vi "CR-导丝上料一致性检测.vi"(8 "error in (no error)":errorcluster caption="错误输入（无错误）", 11 "名称或相对路径":string="Template Program") -> (0 "error in (no error) 2":errorcluster caption="错误输入（无错误）")   [LabVIEW 2017]
uses:
  Picture/SaveButtom.ctl
  <vilib>/vision/Measure.llb/Straight Edge Options.ctl
  <vilib>/vision/Measure.llb/Straight Edge Process.ctl
  <vilib>/vision/Measure.llb/Edge Options.ctl
  <vilib>/vision/Measure.llb/Edge Polarity.ctl
  Global System.vi
  <vilib>/Utility/xml.llb/Write to XML File(string).vi
panel:
  in  "获取图像":bool
  in  "ROI获取":bool
  in  "创建模板":bool
  in  "保存图像":bool
  out "添加的路径":path
  in  "刷新":bool
  in  "测试按钮":bool
  in  "保存按钮":bool
  in  "Main":enum32{"主参数", "模板匹配参数 ", "位置范围设定", "测试效果"}(tab)
  in  "导丝上料一致性基础参数":T1={"IsNorImage"=TRUE, "Exposure Values"=100289, "ImagePath"=path "C:/Users/hedongpo/Desktop/514-hdp/Alignment Assemble System/Test Picture/B/3.bmp"} caption="参数界面" {"Exposure Values" scale=0.0..200000.0}
  in  "导丝上料一致性参数":T7={"Rectangle"={"Left"=0, "Top"=0, "Right"=0, "Bottom"=0, "Rotation"=0.0}, "Find Straight Edge 1"={"Number of Lines"=1, "Type"=enum."First Edge Rake", "Min. Score"=10.0, "Max. Score"=1000.0, "Orientation"=0.0, "Angle Range"=45.0, "Angle Tolerance"=1.0, "Step Size"=11, "Min. SNR (db)"=0.0, "Min. Points (%)"=25.0, "Hough Iterations"=5}, "Process (Edge Detector 1)"=enum."Get All Edges", "Edge Options (Edge Detector 1)"={"Edge Polarity"=0, "Kernel Size"=9, "Width"=1, "Minimum Edge Strength"=8.0, "Interpolation Type"=enum."Bilinear Fixed", "Data Processing Method"=enum."Average"}, "Options (Find Straight Edge 1)"={"Search Direction"=0, "Edge Options"={"Edge Polarity"=0, "Kernel Size"=3, "Width"=1, "Minimum Edge Strength"=32.0, "Interpolation Type"=enum."Bilinear Fixed", "Data Processing Method"=enum."Average"}, "Show Search Area"=TRUE, "Show Search Lines"=TRUE, "Show Edges Found"=TRUE, "Show Result"=TRUE, "Search Area Color"=65280, "Search Lines Color"=255, "Edge Locations Color"=16776960, "Result Color"=16711680, "Overlay Group Name"=""}, "Parameters (Pattern Matching 1)"={"Number of Matches Requested"=1, "Minimum Match Score"=799.0, "Angle Ranges"=[{"Start Angle"=-180.0, "End Angle"=180.0}, {"Start Angle"=0.0, "End Angle"=360.0}]}, "Template File Path (Pattern Matching 1)"=path "D:/Inspect System/Source Code/Template Program/一致性模板.png"} {"Options (Find Straight Edge 1)"."Search Direction" items=["Left to Right", "Right to Left", "Top to Bottom", "Bottom to Top"]; "Options (Find Straight Edge 1)"."Edge Options"."Edge Polarity" items=["All Edges", "Rising Edges", "Falling Edges"]; "Options (Find Straight Edge 1)"."Edge Options"."Minimum Edge Strength" format="%.2f"; "Options (Find Straight Edge 1)"."Edge Options"."Width" step=2; "Options (Find Straight Edge 1)"."Edge Options"."Kernel Size" step=2; "Edge Options (Edge Detector 1)"."Edge Polarity" items=["All Edges", "Rising Edges", "Falling Edges"]; "Find Straight Edge 1"."Min. Points (%)" min=0.0 max=100.0; "Find Straight Edge 1"."Min. SNR (db)" min=0.0; "Find Straight Edge 1"."Max. Score" min=0.0 max=1024.0; "Find Straight Edge 1"."Min. Score" min=0.0 max=1024.0 step=1.0; "Rectangle"."Rotation" format="%.2f"; "Rectangle"."Left" scale=0.0..1024.0; "Rectangle"."Right" scale=0.0..1024.0}
  in  "位置范围设定":T8={"位置1"={"上限"=726.0, "下限"=686.0}, "位置2"={"上限"=874.0, "下限"=834.0}, "位置3"={"上限"=997.0, "下限"=957.0}, "位置4"={"上限"=1139.0, "下限"=1099.0}, "位置5"={"上限"=1283.0, "下限"=1243.0}, "位置6"={"上限"=1429.0, "下限"=1389.0}, "位置7"={"上限"=1576.0, "下限"=1536.0}, "位置8"={"上限"=1728.0, "下限"=1688.0}, "位置9"={"上限"=1879.0, "下限"=1839.0}, "位置10"={"上限"=2036.0, "下限"=1996.0}}
  out "原始图像":T9(plugin-control)
  out "模板图片":T9(plugin-control)
  out "一致性结果字符串":string
  out "数字":i32
  out "动态范围":sgl[](array[numeric])
  out "路径输出":path
  in  "Vision Paramter Save Buttom":T10
  out "system time":string
  in  "取消按钮":bool
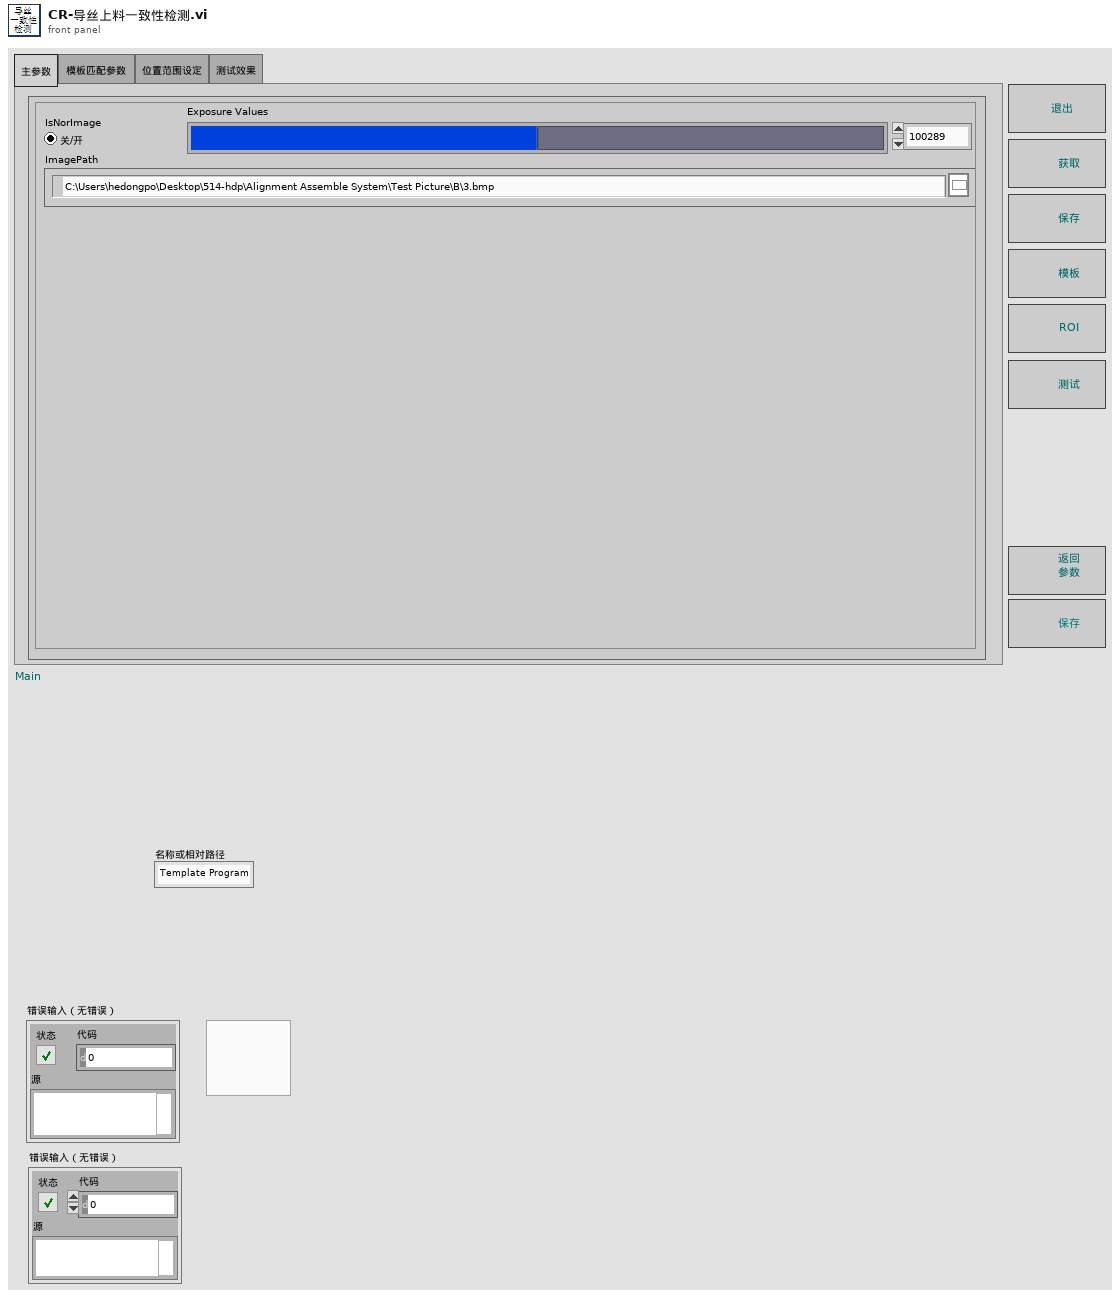
[diagram p1: front panel]
types:
  T1 = cluster{"IsNorImage":bool, "Exposure Values":u32, "ImagePath":path}
  T2 = typedef "IMAQ Rectangle" = cluster{"Left":i32, "Top":i32, "Right":i32, "Bottom":i32, "Rotation":dbl}
  T3 = typedef "Straight Edge Options.ctl" = cluster{"Number of Lines":i32, "Type":T4, "Min. Score":dbl, "Max. Score":dbl, "Orientation":dbl, "Angle Range":dbl, "Angle Tolerance":dbl, "Step Size":u32, "Min. SNR (db)":dbl, "Min. Points (%)":dbl, "Hough Iterations":i32}
  T4 = typedef "Straight Edge Process.ctl" = enum32{"First Edge Rake", "Best Edge Rake", "Hough Edge Rake", "First Edge Projection", "Best Edge Projection"}
  T5 = typedef "Edge Options.ctl" = cluster{"Edge Polarity":T6, "Kernel Size":u32, "Width":u32, "Minimum Edge Strength":sgl, "Interpolation Type":enum32{"Zero Order", "Bilinear", "Quadratic", "Cubic", "Bilinear Fixed"}, "Data Processing Method":enum32{"Average", "Median"}}
  T6 = typedef "Edge Polarity.ctl" = u32
  T7 = cluster{"Rectangle":T2, "Find Straight Edge 1":T3, "Process (Edge Detector 1)":enum16{"Get First Edge", "Get First + Last Edge", "Get All Edges", "Get Best Edge"}, "Edge Options (Edge Detector 1)":cluster{"Edge Polarity":u32, "Kernel Size":u32, "Width":u32, "Minimum Edge Strength":sgl, "Interpolation Type":enum32{"Zero Order", "Bilinear", "Quadratic", "Cubic", "Bilinear Fixed"}, "Data Processing Method":enum32{"Average", "Median"}}, "Options (Find Straight Edge 1)":cluster{"Search Direction":u32, "Edge Options":T5, "Show Search Area":bool, "Show Search Lines":bool, "Show Edges Found":bool, "Show Result":bool, "Search Area Color":u32, "Search Lines Color":u32, "Edge Locations Color":u32, "Result Color":u32, "Overlay Group Name":string}, "Parameters (Pattern Matching 1)":cluster{"Number of Matches Requested":i32, "Minimum Match Score":sgl, "Angle Ranges":cluster{"Start Angle":sgl, "End Angle":sgl}[]}, "Template File Path (Pattern Matching 1)":path}
  T8 = cluster{"位置1":cluster{"上限":dbl, "下限":dbl}, "位置2":cluster{"上限":dbl, "下限":dbl}, "位置3":cluster{"上限":dbl, "下限":dbl}, "位置4":cluster{"上限":dbl, "下限":dbl}, "位置5":cluster{"上限":dbl, "下限":dbl}, "位置6":cluster{"上限":dbl, "下限":dbl}, "位置7":cluster{"上限":dbl, "下限":dbl}, "位置8":cluster{"上限":dbl, "下限":dbl}, "位置9":cluster{"上限":dbl, "下限":dbl}, "位置10":cluster{"上限":dbl, "下限":dbl}}
  T9 = typedef "IMAQ Image.ctl" = refnum<image>
  T10 = typedef "SaveButtom.ctl" = bool
  T11 = cluster{"index":i32, "this vi":refnum<vi>, "error out":errorcluster}
  T12 = cluster{"master data":string, "priority":u16, "secondary data":string[]}
  T13 = cluster{"case name":string[], "queue array":refnum<queue>[]}
  T14 = typedef "Image Type" = u32
  T15 = typedef "IMAQdx.ctl" = refnum<k21>
  T16 = cluster{"Global Rectangle":i32[], "Contours":cluster{"Contour Type":u32, "ROI Type":u32, "Points":i32[]}[]}
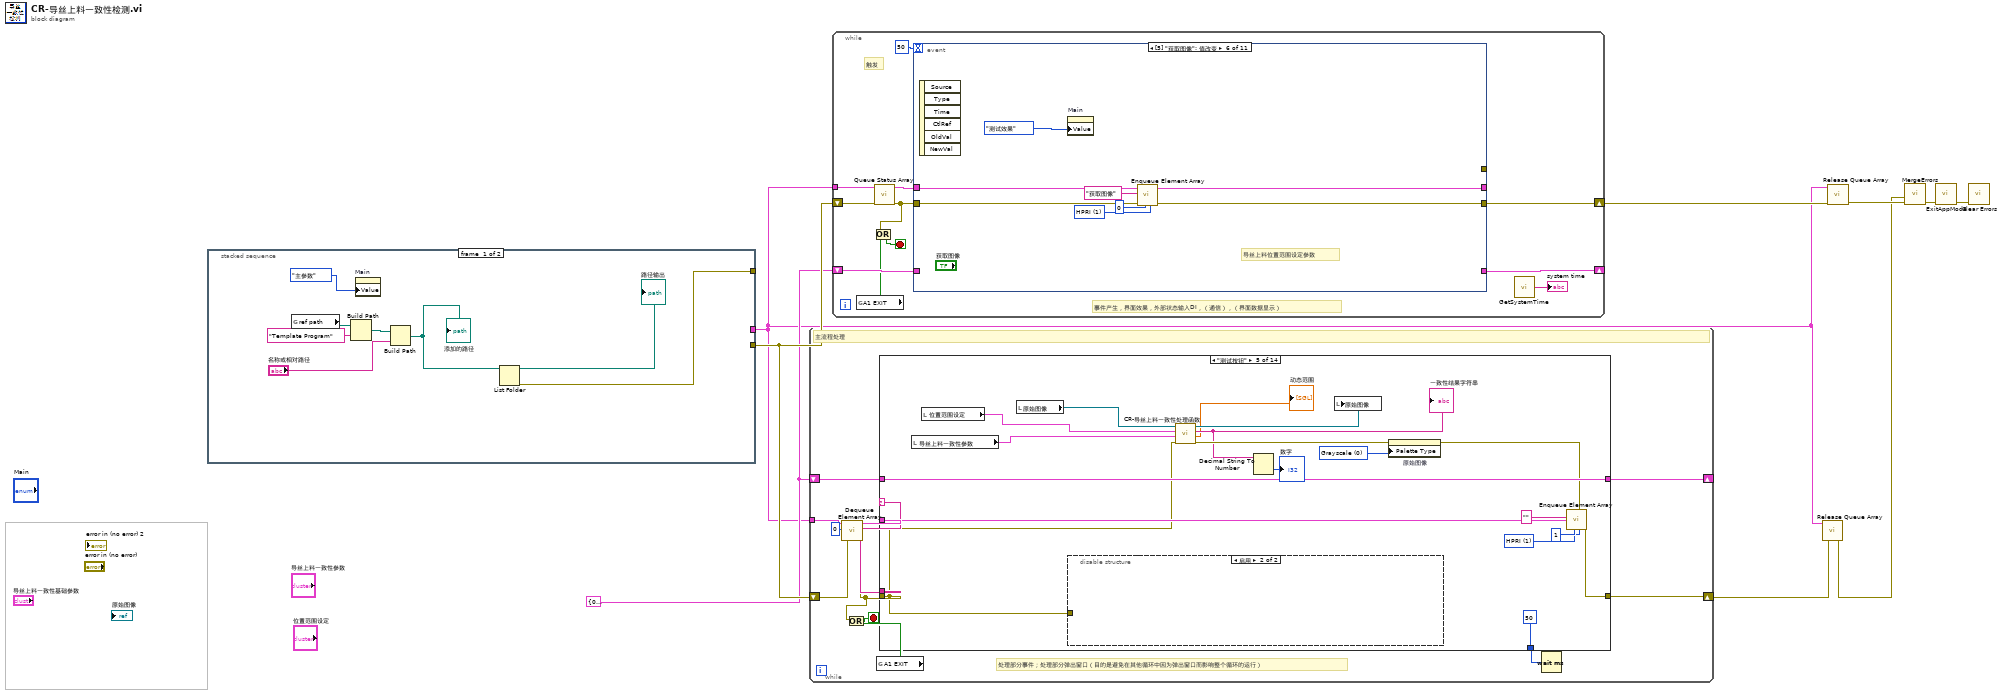
[diagram p0: block diagram]
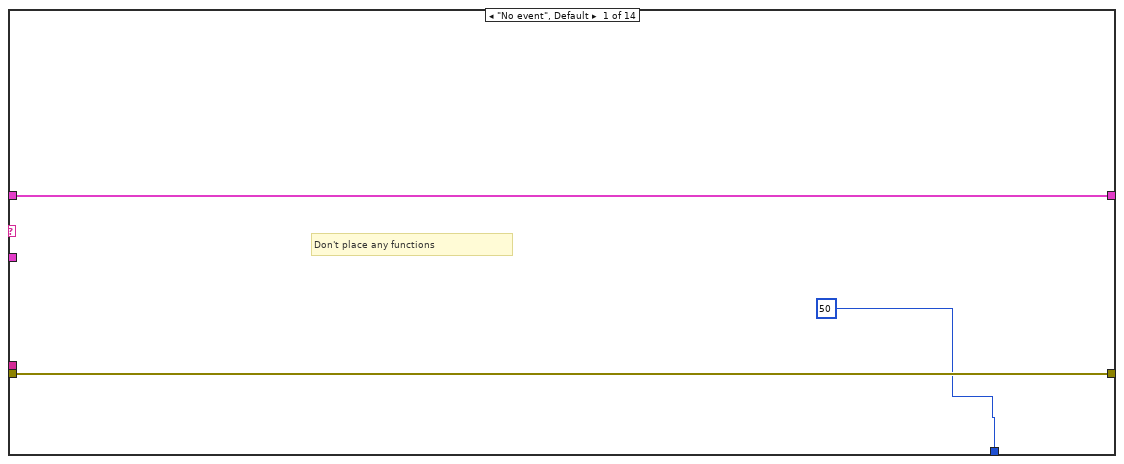
[diagram p2: hidden frame]
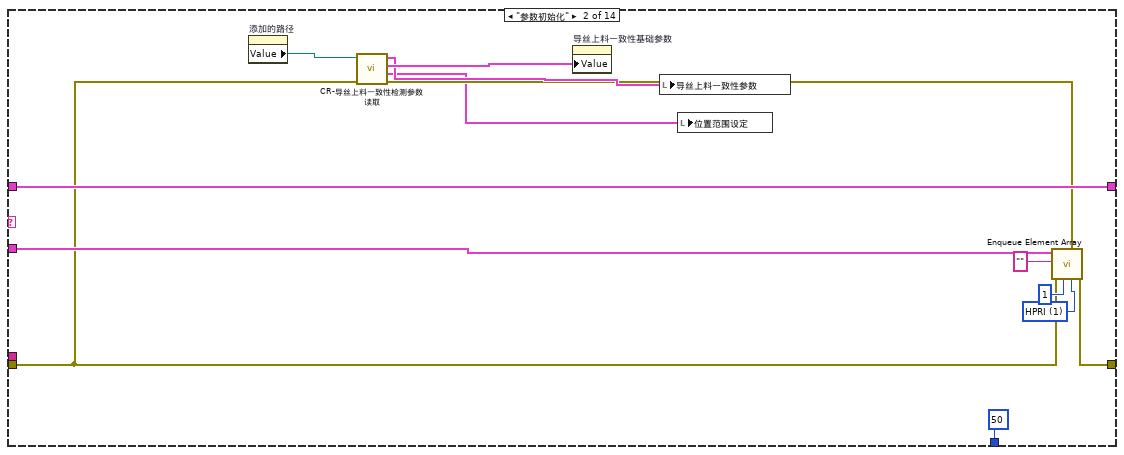
[diagram p3: hidden frame]
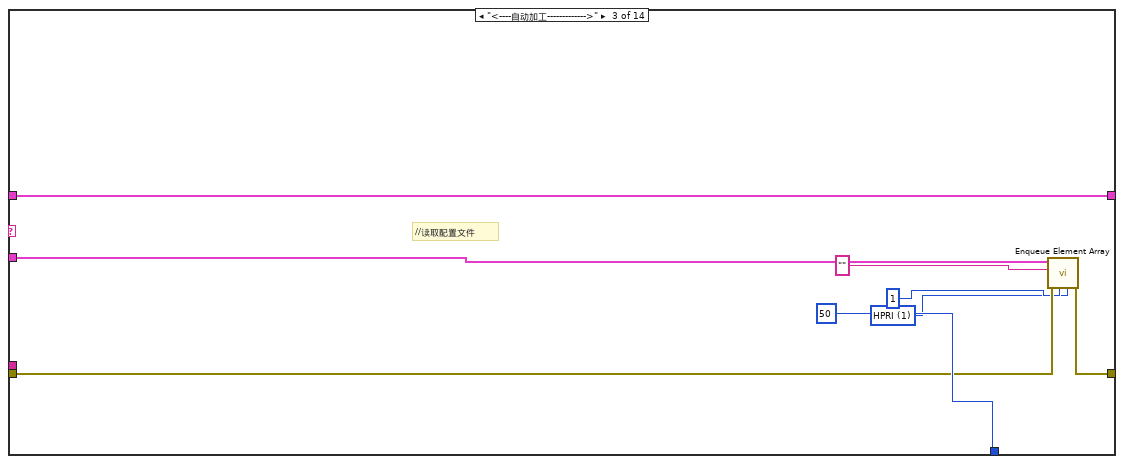
[diagram p4: hidden frame]
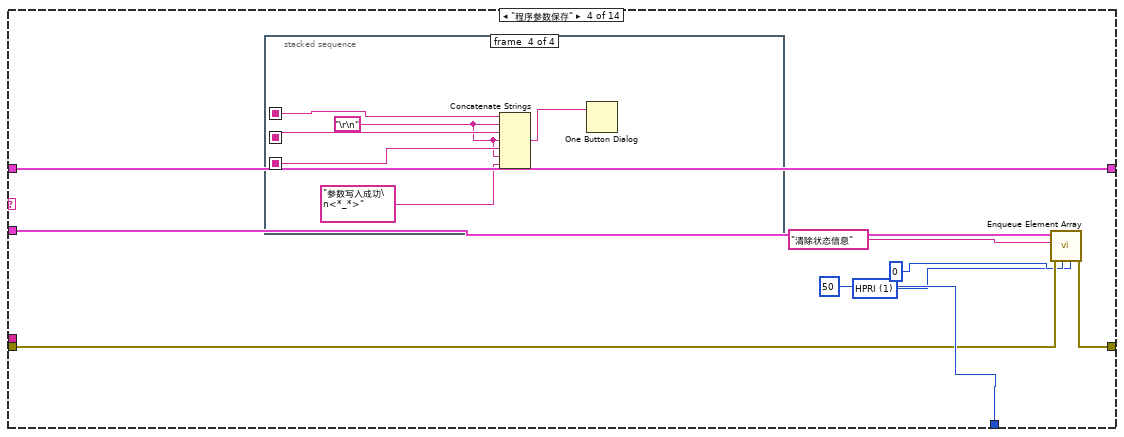
[diagram p5: hidden frame]
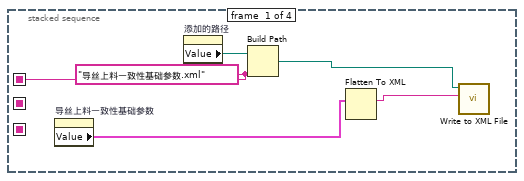
[diagram p6: hidden frame]
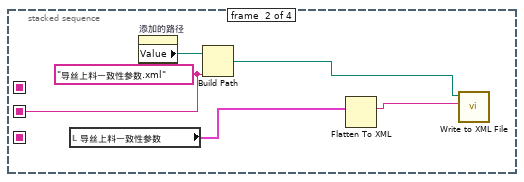
[diagram p7: hidden frame]
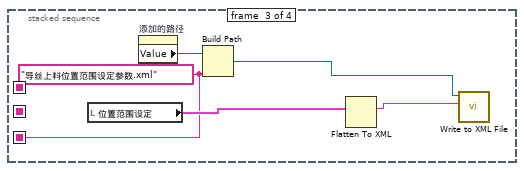
[diagram p8: hidden frame]
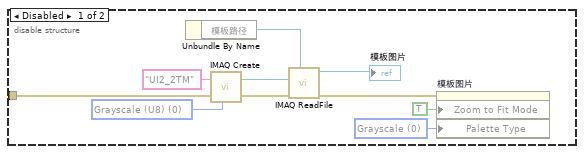
[diagram p9: hidden frame]
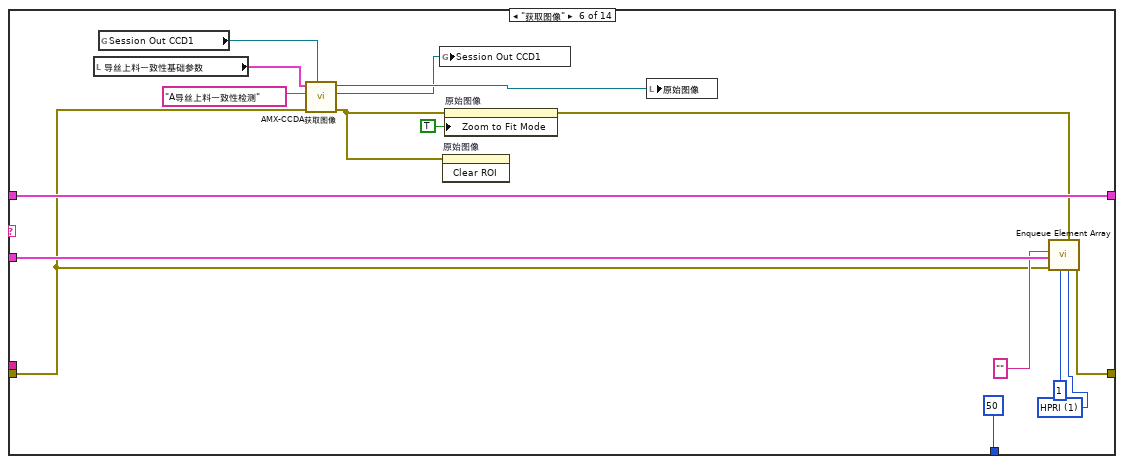
[diagram p10: hidden frame]
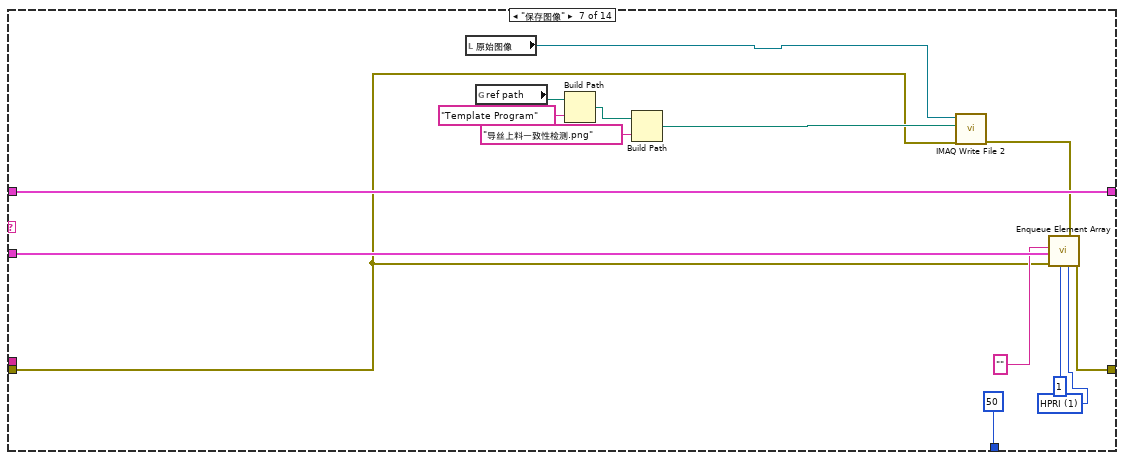
[diagram p11: hidden frame]
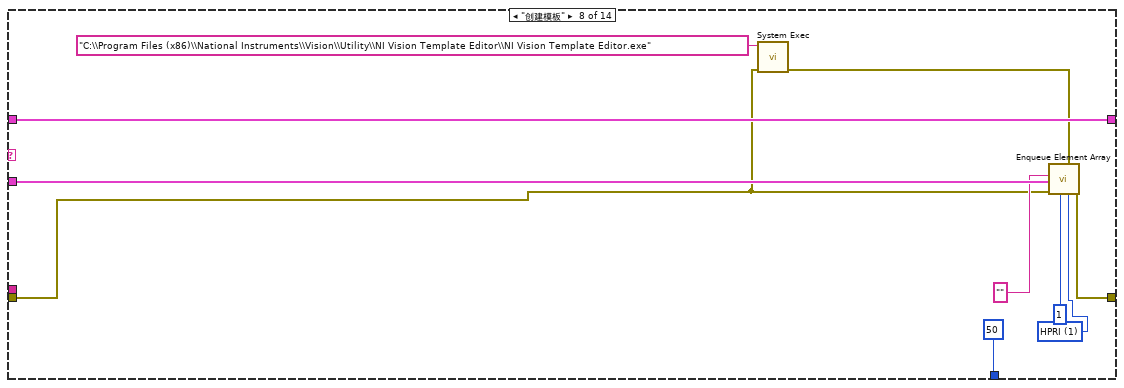
[diagram p12: hidden frame]
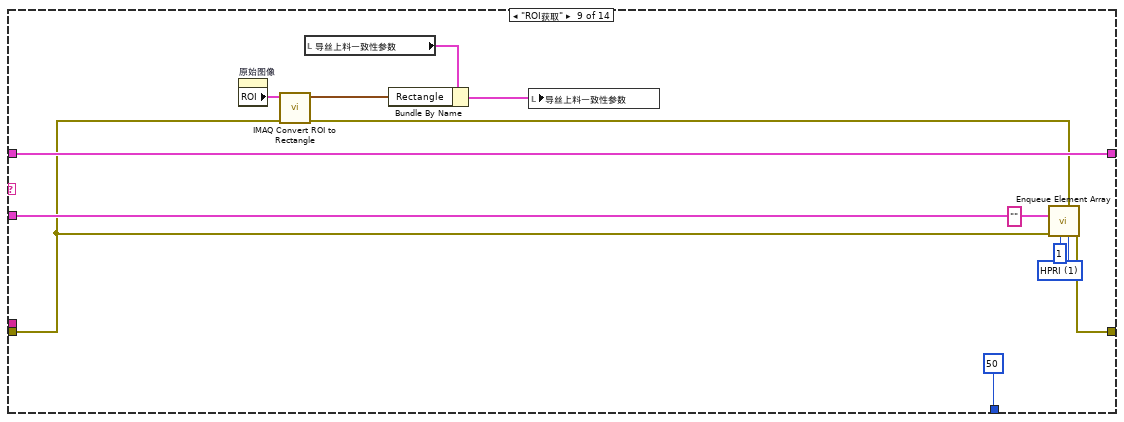
[diagram p13: hidden frame]
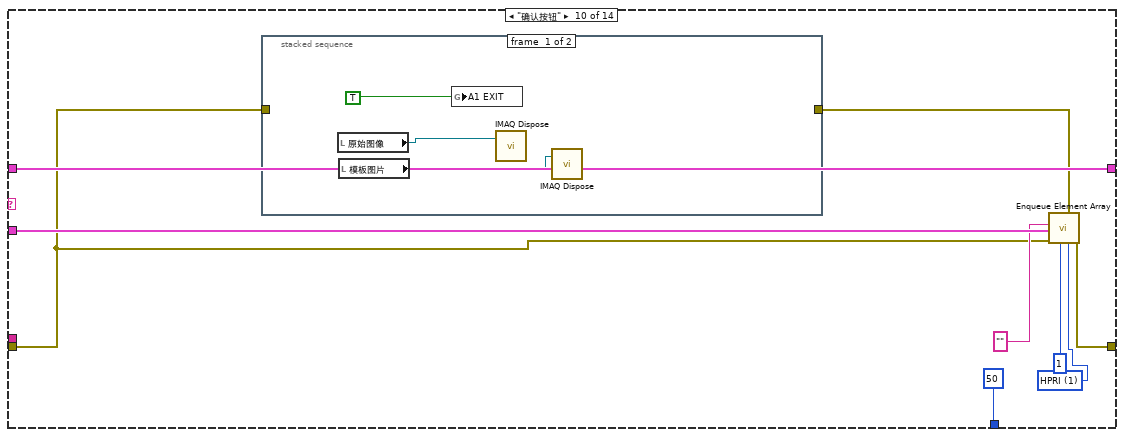
[diagram p14: hidden frame]
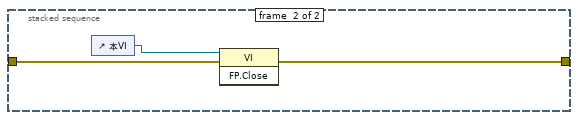
[diagram p15: hidden frame]
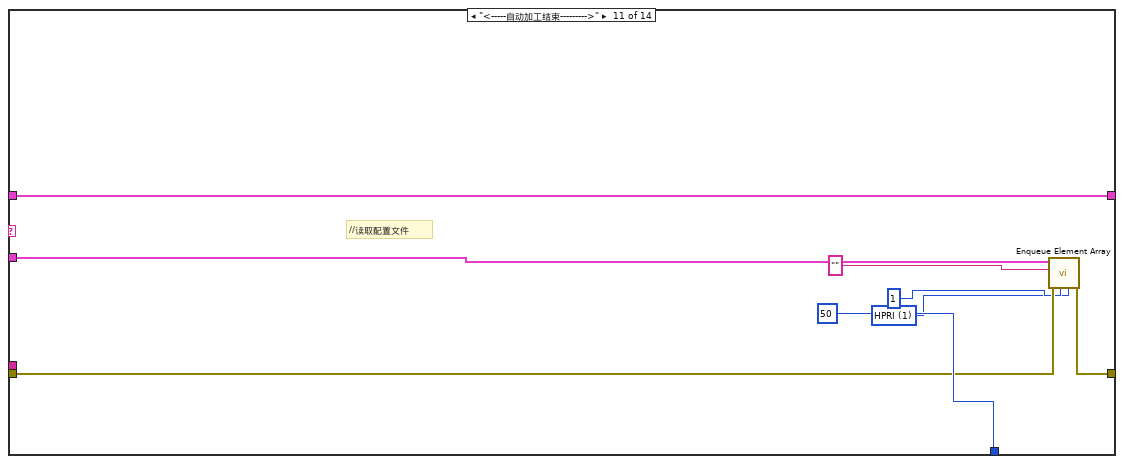
[diagram p16: hidden frame]
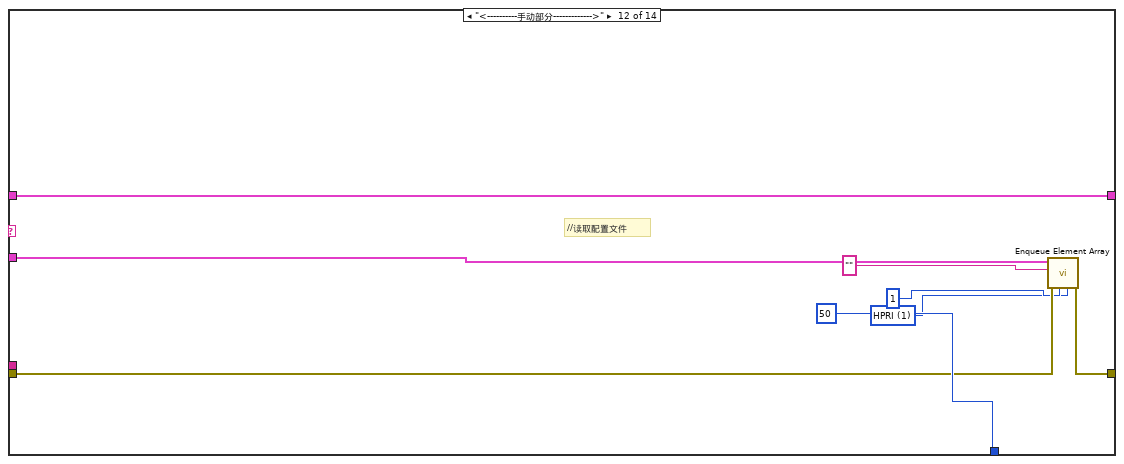
[diagram p17: hidden frame]
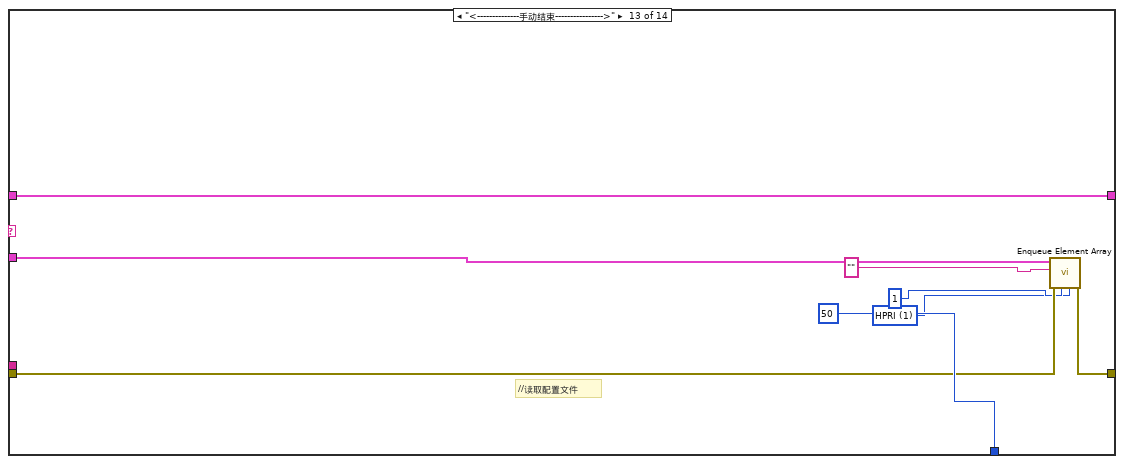
[diagram p18: hidden frame]
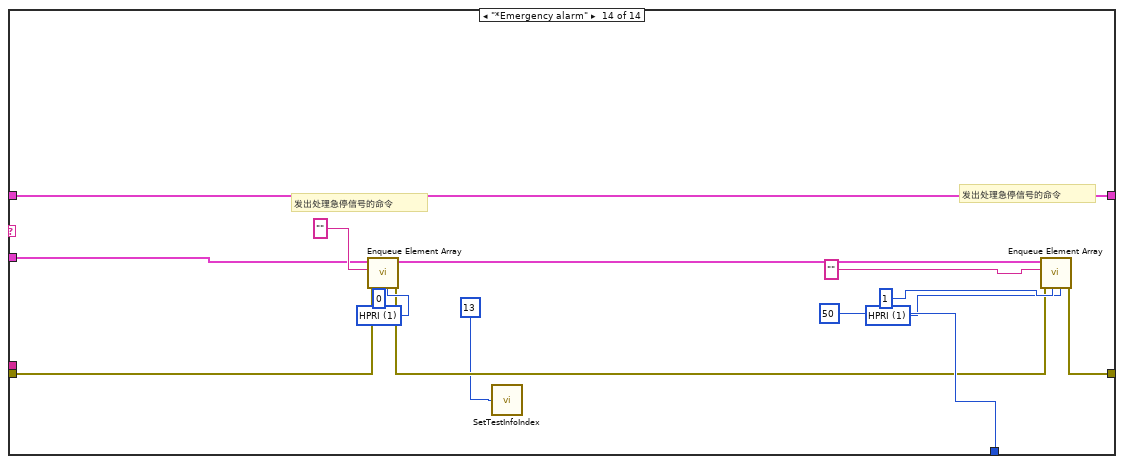
[diagram p19: hidden frame]
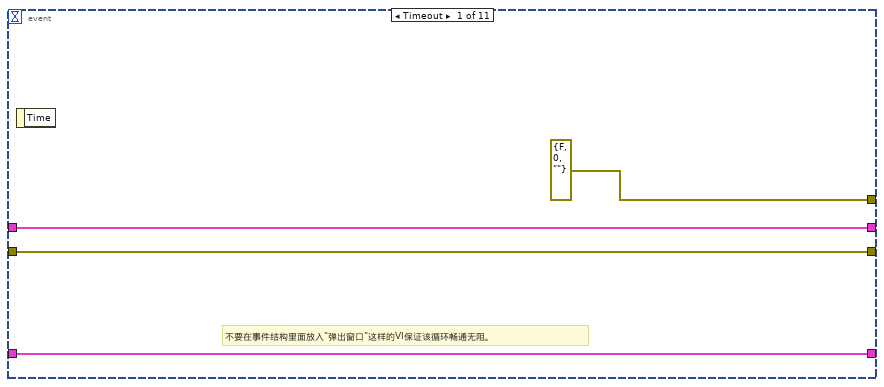
[diagram p20: hidden frame]
diagram:
  w4 = T11 {"index"=0, "this vi"=refnum, "error out"={"status"=FALSE, "code"=0, "source"=""}} ("parameter buffer")
  n1 = stacked-sequence {
    tunnel: [w15 _] -> _
    tunnel: [_ w19] -> w5
    tunnel: [_ w18] -> w1
    frame #0 {
      n2 = global read "Global System.vi" "ref path"() -> (w13:path)
      n3 = Build Path(base path=w13, name or relative path="Template Program" ("名称或相对路径")) -> (appended path=w11:path)
      n4 = property on="Main" class="TabCtl (严格)"("Value"=enum32{"主参数", "模板匹配参数 ", "位置范围设定", "测试效果"}."主参数" ("Main")) -> ()  [unwired: 2 in, 2 out]
      n5 = Build Path(base path=w11, name or relative path="名称或相对路径") -> (appended path=w17:path)
      "添加的路径" <- w17
      n6 = List Folder(path=w17) -> (path out=→"路径输出":path, error out=w15:errorcluster)  [unwired: 3 in, 2 out]
    }
    frame #1 {
      w27 = string[] ["comm queue1", "data queue 11", "data queue 12", "data queue 13", "data queue 14"]  # queue name
      w28 = 4  # queue num
      w29 = T12 {"master data"="", "priority"=0, "secondary data"=[]}  # element data type
      n7 = call "Obtain Queue Array.vi"("queue name"=w27, "element data type"=w29, "queue num"=w28) -> ("error out"=w23:errorcluster, "queue out"=w24:T13)  [unwired: 2 in, 1 out]
      n8 = call "Enqueue Element Array.vi"("queue index"=0, "error in"=w23, "master data"="参数初始化", "queue in"=w24) -> ("error out"=w22:errorcluster, "queue out"=w21:T13)  [unwired: 6 in]
      n9 = disable-structure shown="启用" {
        disable-tunnel: w22 -> [w35 w36]
        disable-tunnel: w21 -> [w34 w37]
        disable-tunnel: "Loading Variable" ("master data") -> [w33 _]
        disable-tunnel: [w31 w36] -> w19
        disable-tunnel: [w30 w37] -> w18
        frame Disabled {
          n10 = call "Enqueue Element Array.vi"("queue index"=12, "error in"=w35, "master data"=w33, "queue in"=w34) -> ("error out"=w31:errorcluster, "queue out"=w30:T13)  [unwired: 6 in]
        }
        frame Enabled {
        }
      }
    }
  }
  n11 = while {
    shift-right: [w50] -> w3
    shift-left: w5 -> [w41]
    shift-right: [w47] -> _
    shift-left: w4 -> [w48]
    tunnel: w1 -> [w43]
    stop <- w38 stop-if-true
    # "处理部分事件；处理部分弹出窗口（目的是避免在其他循环中因为弹出窗口而影响整个循环的运行）"
    # "主流程处理"
    n12 = call "Dequeue Element Array.vi"("queue in"=w43, "queue index"=0, "error in"=w41) -> ("queue out"=w46:T13, "master data"=w45:string, "secondary data"=w44:string[], "error out"=w40:errorcluster)  [unwired: 2 in, 1 out]
    n13 = global read "Global System.vi" "A1 EXIT"() -> (w39:bool)
    n14 = Or(x=w40, y=w39) -> (x .or. y?=w38:bool)
    n15 = case shown="\"测试按钮\"" w45 {
      tunnel: w46 -> [_ w65 w73 w75 w120 w146 w161 w171 w184 w193 w207 w215 w223 w229]
      tunnel: w40 -> [w52 w58 w69 w79 w114 w138 w148 w164 w177 w187 w203 w211 w219 w226]
      tunnel: [w52 w64 w72 w81 w119 w145 w160 w170 w183 w192 w206 w214 w222 w237] -> w50
      tunnel: [50 50 50 50 50 50 50 50 50 50 50 50 50 50] -> w49
      tunnel: w48 -> [w53 w60 w70 w76 w115 w141 w156 w166 w179 w188 w204 w212 w220 w235]
      tunnel: [w53 w60 w70 w76 w115 w141 w156 w166 w179 w188 w204 w212 w220 w235] -> w47
      tunnel: w44 -> [_ _ _ _ _ _ _ _ _ _ _ _ _ _]
      frame "No event", Default {
        # "Don't place any functions"
      }
      frame "参数初始化" {
        w61 = u16 1 items=["HPRI"=1, "LPRI"=0] ("priority")
        n16 = property on="添加的路径" class="Path"() -> ("Value"=w59:path)  [unwired: 2 in, 2 out]
        n17 = call "CR-导丝上料一致性检测参数读取.vi"("error in (no error)"=w58, "基路径"=w59) -> ("error out"=w55:errorcluster, "CR位置范围设定"=w54:T8, "导丝上料一致性基础参数"=w57:T1, "CR导丝上料一致性参数"=w56:T7)  [unwired: 5 in]
        n18 = property on="导丝上料一致性基础参数" class="Clust (严格)"("Value"=w57) -> ()  [unwired: 2 in, 2 out]
        n19 = local write "导丝上料一致性参数"(w56) -> ()
        n20 = local write "位置范围设定"(w54) -> ()
        n21 = call "Enqueue Element Array.vi"("priority"=w61, "device error in"=w55, "queue index"=1, "error in"=w58, "master data"="" ("Element 1"), "queue in"=w65) -> ("error out"=w64:errorcluster)  [unwired: 4 in, 1 out]
      }
      frame "<----自动加工------------->" {
        w67 = u16 1 items=["HPRI"=1, "LPRI"=0] ("priority")
        # "//读取配置文件"
        n22 = call "Enqueue Element Array.vi"("priority"=w67, "queue index"=1, "error in"=w69, "master data"="" ("Element 1"), "queue in"=w73) -> ("error out"=w72:errorcluster)  [unwired: 5 in, 1 out]
      }
      frame "程序参数保存" {
        w77 = u16 1 items=["HPRI"=1, "LPRI"=0] ("priority")
        n23 = stacked-sequence {
          seq-local: [w83 _ _ _] -> [_ _ _ w102]
          seq-local: [_ w89 _ _] -> [_ _ _ w100]
          seq-local: [_ _ w93 _] -> [_ _ _ w99]
          frame #0 {
            w83 = "导丝上料一致性基础参数.xml" ("名称或相对路径")
            n24 = property on="导丝上料一致性基础参数" class="Clust (严格)"() -> ("Value"=w86:T1)  [unwired: 2 in, 2 out]
            n25 = property on="添加的路径" class="Path"() -> ("Value"=w87:path)  [unwired: 2 in, 2 out]
            n26 = Build Path(base path=w87, name or relative path=w83) -> (appended path=w84:path)
            n27 = Flatten To XML(anything=w86) -> (xml string=w85:string)
            n28 = call-poly <vilib>:"Write to XML File.vi"("XML Input"=w85, "XML File Path"=w84) -> ()  [unwired: 7 in, 3 out]
          }
          frame #1 {
            w89 = "导丝上料一致性参数.xml" ("名称或相对路径")
            n29 = local read "导丝上料一致性参数"() -> (w88:T7)
            n30 = property on="添加的路径" class="Path"() -> ("Value"=w92:path)  [unwired: 2 in, 2 out]
            n31 = Build Path(base path=w92, name or relative path=w89) -> (appended path=w90:path)
            n32 = Flatten To XML(anything=w88) -> (xml string=w91:string)
            n33 = call-poly <vilib>:"Write to XML File.vi"("XML Input"=w91, "XML File Path"=w90) -> ()  [unwired: 7 in, 3 out]
          }
          frame #2 {
            w93 = "导丝上料位置范围设定参数.xml" ("名称或相对路径")
            n34 = local read "位置范围设定"() -> (w94:T8)
            n35 = property on="添加的路径" class="Path"() -> ("Value"=w97:path)  [unwired: 2 in, 2 out]
            n36 = Build Path(base path=w97, name or relative path=w93) -> (appended path=w95:path)
            n37 = Flatten To XML(anything=w94) -> (xml string=w96:string)
            n38 = call-poly <vilib>:"Write to XML File.vi"("XML Input"=w96, "XML File Path"=w95) -> ()  [unwired: 7 in, 3 out]
          }
          frame #3 {
            w98 = "\r\n"
            n39 = Concatenate Strings(w102, w98, w100, w98, w99, w98, "参数写入成功\n<*_*>" ("消息")) -> (w101:string)
            n40 = One Button Dialog(message=w101) -> ()  [unwired: 1 in, 1 out]
          }
        }
        n41 = call "Enqueue Element Array.vi"("priority"=w77, "queue index"=0, "error in"=w79, "master data"="清除状态信息" ("Element 1"), "queue in"=w75) -> ("error out"=w81:errorcluster)  [unwired: 5 in, 1 out]
      }
      frame "测试按钮" {
        w110 = u32 0 items=["Grayscale", "Binary", "Gradient", "Rainbow", "Temperature", "User Defined", "Binary 16 Bit", "Gradient 16 Bit", "Rainbow 16 Bit", "Temperature 16 Bit", "User Defined 16 Bit"] ("Palette:Palette Type")
        w116 = u16 1 items=["HPRI"=1, "LPRI"=0] ("priority")
        n42 = local read "导丝上料一致性参数"() -> (w107:T7)
        n43 = local read "位置范围设定"() -> (w108:T8)
        n44 = local read "原始图像"() -> (w112:T9)
        n45 = disable-structure shown="启用" {
          disable-tunnel: w114 -> [w131 _]
          frame Disabled {
            w123 = u32 0 items=["Grayscale", "Binary", "Gradient", "Rainbow", "Temperature", "User Defined", "Binary 16 Bit", "Gradient 16 Bit", "Rainbow 16 Bit", "Temperature 16 Bit", "User Defined 16 Bit"] ("Palette:Palette Type")
            w129 = T14 0 items=["Grayscale (U8)", "Grayscale (I16)", "Grayscale (SGL)", "Complex (CSG)", "RGB (U32)", "HSL (U32)", "RGB (U64)", "Grayscale (U16)"] ("Image Type")
            n46 = Unbundle By Name() -> ("模板路径"=w122:path)  [unwired: 1 in]
            n47 = call "IMAQ Create"("Image Name"="UI2_2TM", "Image Type"=w129, "error in (no error)"=w131) -> ("New Image"=w128:T9, "error out"=w127:errorcluster)  [unwired: 2 in]
            n48 = call "IMAQ ReadFile"("File Path"=w122, "error in (no error)"=w127, "Image"=w128) -> ("error out"=w125:errorcluster, "Image Out"=→"模板图片":T9)  [unwired: 4 in, 3 out]
            n49 = property on="模板图片" class="ImageControl"(error in=w125, "Zoom to Fit Mode"=TRUE, "Palette Type"=w123) -> ()  [unwired: 1 in, 2 out]
          }
          frame Enabled {
          }
        }
        n50 = call "CR-导丝上料一致性处理函数.vi"("error in (no error)"=w114, "导丝上料一致性参数"=w107, "位置范围设定"=w108, "Image in"=w112) -> ("error out"=w111:errorcluster, "动态范围"=→"动态范围":sgl[], "一致性结果字符串"=w106:string, "Image out"=w113:T9)  [unwired: 4 in]
        "一致性结果字符串" <- w106
        n51 = Decimal String To Number(string=w106) -> (number=→"数字":i32)  [unwired: 2 in, 1 out]
        n52 = local write "原始图像"(w113) -> ()
        n53 = property on="原始图像" class="ImageControl"(error in=w111, "Palette Type"=w110) -> (error out=w109:errorcluster)  [unwired: 1 in, 1 out]
        n54 = call "Enqueue Element Array.vi"("priority"=w116, "device error in"=w109, "queue index"=1, "master data"="" ("Element 1"), "queue in"=w120) -> ("error out"=w119:errorcluster)  [unwired: 5 in, 1 out]
      }
      frame "获取图像" {
        w142 = u16 1 items=["HPRI"=1, "LPRI"=0] ("priority")
        n55 = local read "导丝上料一致性基础参数"() -> (w132:T1)
        n56 = global read "Global System.vi" "Session Out CCD1"() -> (w134:T15)
        n57 = call "AMX-CCDA获取图像.vi"("Session Out CCD2"=w134, "error in (no error)"=w138, "Image Name"="A导丝上料一致性检测", "ParamsUI"=w132) -> ("error out"=w135:errorcluster, "Session Out"=w133:T15, "Image out"=w139:T9)  [unwired: 4 in, 1 out]
        n58 = global write "Global System.vi" "Session Out CCD1"(w133) -> ()
        n59 = invoke on="原始图像" class="ImageControl" method="Clear ROI"(error in=w135) -> ()  [unwired: 2 in, 3 out]
        n60 = property on="原始图像" class="ImageControl"(error in=w135, "Zoom to Fit Mode"=TRUE) -> (error out=w136:errorcluster)  [unwired: 1 in, 1 out]
        n61 = local write "原始图像"(w139) -> ()
        n62 = call "Enqueue Element Array.vi"("priority"=w142, "device error in"=w136, "queue index"=1, "error in"=w138, "master data"="" ("Element 1"), "queue in"=w146) -> ("error out"=w145:errorcluster)  [unwired: 4 in, 1 out]
      }
      frame "保存图像" {
        w157 = u16 1 items=["HPRI"=1, "LPRI"=0] ("priority")
        n63 = local read "原始图像"() -> (w149:T9)
        n64 = global read "Global System.vi" "ref path"() -> (w155:path)
        n65 = Build Path(base path=w155, name or relative path="Template Program" ("名称或相对路径")) -> (appended path=w153:path)
        n66 = Build Path(base path=w153, name or relative path="导丝上料一致性检测.png" ("名称或相对路径")) -> (appended path=w151:path)
        n67 = call-poly "IMAQ Write File 2"("error in (no error)"=w148, "File Path"=w151, "Image"=w149) -> ("error out"=w150:errorcluster)  [unwired: 7 in, 1 out]
        n68 = call "Enqueue Element Array.vi"("priority"=w157, "device error in"=w150, "queue index"=1, "error in"=w148, "master data"="" ("Element 1"), "queue in"=w161) -> ("error out"=w160:errorcluster)  [unwired: 4 in, 1 out]
      }
      frame "创建模板" {
        w167 = u16 1 items=["HPRI"=1, "LPRI"=0] ("priority")
        n69 = call <vilib>:"System Exec.vi"("error in (no error)"=w164, "command line"="C:\\Program Files (x86)\\National Instruments\\Vision\\Utility\\NI Vision Template Editor\\NI Vision Template Editor.exe") -> ("error out"=w163:errorcluster)  [unwired: 6 in, 3 out]
        n70 = call "Enqueue Element Array.vi"("priority"=w167, "device error in"=w163, "queue index"=1, "error in"=w164, "master data"="" ("Element 1"), "queue in"=w171) -> ("error out"=w170:errorcluster)  [unwired: 4 in, 1 out]
      }
      frame "ROI获取" {
        w180 = u16 1 items=["HPRI"=1, "LPRI"=0] ("priority")
        n71 = property on="原始图像" class="ImageControl"() -> ("ROI"=w178:T16)  [unwired: 2 in, 2 out]
        n72 = call "IMAQ Convert ROI to Rectangle"("error in (no error)"=w177, "ROI Descriptor"=w178) -> ("error out"=w173:errorcluster, "Rectangle"=w175:T2)  [unwired: 7 in]
        n73 = local read "导丝上料一致性参数"() -> (w176:T7)
        n74 = Bundle By Name(cluster=w176, "Rectangle"=w175) -> (w174:T7)
        n75 = local write "导丝上料一致性参数"(w174) -> ()
        n76 = call "Enqueue Element Array.vi"("priority"=w180, "device error in"=w173, "queue index"=1, "error in"=w177, "master data"="" ("Element 1"), "queue in"=w184) -> ("error out"=w183:errorcluster)  [unwired: 4 in, 1 out]
      }
      frame "确认按钮" {
        w189 = u16 1 items=["HPRI"=1, "LPRI"=0] ("priority")
        n77 = stacked-sequence {
          tunnel: w187 -> [_ w199]
          tunnel: [_ w198] -> w186
          frame #0 {
            n78 = local read "原始图像"() -> (w196:T9)
            n79 = local read "模板图片"() -> (w195:T9)
            n80 = global write "Global System.vi" "A1 EXIT"(TRUE ("EXIT")) -> ()
            n81 = call "IMAQ Dispose"("Image"=w196) -> ()  [unwired: 5 in, 1 out]
            n82 = call "IMAQ Dispose"("Image"=w195) -> ()  [unwired: 5 in, 1 out]
          }
          frame #1 {
            n83 = control-ref of="本VI"() -> (w200:refnum<vi>)
            n84 = invoke class="VI" method="FP.Close"(reference=w200, error in=w199) -> (error out=w198:errorcluster)  [unwired: 1 in, 2 out]
          }
        }
        n85 = call "Enqueue Element Array.vi"("priority"=w189, "device error in"=w186, "queue index"=1, "error in"=w187, "master data"="" ("Element 1"), "queue in"=w193) -> ("error out"=w192:errorcluster)  [unwired: 4 in, 1 out]
      }
      frame "<-----自动加工结束--------->" {
        w201 = u16 1 items=["HPRI"=1, "LPRI"=0] ("priority")
        # "//读取配置文件"
        n86 = call "Enqueue Element Array.vi"("priority"=w201, "queue index"=1, "error in"=w203, "master data"="" ("Element 1"), "queue in"=w207) -> ("error out"=w206:errorcluster)  [unwired: 5 in, 1 out]
      }
      frame "<----------手动部分------------->" {
        w209 = u16 1 items=["HPRI"=1, "LPRI"=0] ("priority")
        # "//读取配置文件"
        n87 = call "Enqueue Element Array.vi"("priority"=w209, "queue index"=1, "error in"=w211, "master data"="" ("Element 1"), "queue in"=w215) -> ("error out"=w214:errorcluster)  [unwired: 5 in, 1 out]
      }
      frame "<--------------手动结束---------------->" {
        w217 = u16 1 items=["HPRI"=1, "LPRI"=0] ("priority")
        # "//读取配置文件"
        n88 = call "Enqueue Element Array.vi"("priority"=w217, "queue index"=1, "error in"=w219, "master data"="" ("Element 1"), "queue in"=w223) -> ("error out"=w222:errorcluster)  [unwired: 5 in, 1 out]
      }
      frame "*Emergency alarm" {
        w232 = u16 1 items=["HPRI"=1, "LPRI"=0] ("priority")
        w233 = u16 1 items=["HPRI"=1, "LPRI"=0] ("priority")
        # "发出处理急停信号的命令"
        # "发出处理急停信号的命令"
        n89 = call "Enqueue Element Array.vi"("priority"=w232, "queue index"=0, "error in"=w226, "master data"="" ("Element 1"), "queue in"=w229) -> ("error out"=w227:errorcluster, "queue out"=w228:T13)  [unwired: 5 in]
        n90 = call "SetTestInfoIndex.vi"("test info index"=13) -> ()
        n91 = call "Enqueue Element Array.vi"("priority"=w233, "queue index"=1, "error in"=w227, "master data"="" ("Element 1"), "queue in"=w228) -> ("error out"=w237:errorcluster)  [unwired: 5 in, 1 out]
      }
    }
    n92 = Wait (ms)(milliseconds to wait=w49) -> ()  [unwired: 1 out]
  }
  n93 = while {
    shift-right: [w242] -> w6
    shift-left: w5 -> [w246]
    shift-right: [w244] -> _
    shift-left: w4 -> [w245]
    tunnel: w1 -> [w248]
    stop <- w239 stop-if-true
    # "触发"
    # "事件产生，界面效果，外部状态输入DI，（通信），（界面数据显示）"
    n94 = global read "Global System.vi" "A1 EXIT"() -> (w240:bool)
    n95 = call "Queue Status Array.vi"("error in (no error)"=w246, "queue in"=w248) -> ("error out"=w241:errorcluster, "queue out"=w243:T13)  [unwired: 4 in]
    n96 = Or(x=w241, y=w240) -> (x .or. y?=w239:bool)
    n97 = event shown="[5] \"获取图像\": 值改变" {
      selector: _ -> [_ _ _ _ _ _ _ _ _ _ _]
      dyn-events: _ -> [_ _ _ _ _ _ _ _ _ _ _]
      timeout: 50 -> [_ _ _ _ _ _ _ _ _ _ _]
      tunnel: w245 -> [w253 w261 _ _ _ _ _ _ _ _ _]
      tunnel: [w253 w261 _ _ _ _ _ _ _ _ _] -> w244
      tunnel: [errorcluster {"status"=FALSE, "code"=0, "source"=""} ("error out") _ _ _ _ _ _ _ _ _ _] -> _
      tunnel: w243 -> [w251 w260 w266 w273 w280 w288 w295 w302 w310 w318 w326]
      tunnel: w241 -> [w250 w259 w265 w272 w279 w287 w294 w301 w309 w317 w325]
      tunnel: [w250 w258 w263 w270 w277 w285 w292 w299 w307 w315 w323] -> w242
      tunnel: [w251 w257 w264 w271 w278 w286 w293 w300 w308 w316 w324] -> _
      event Timeout {
        # "不要在事件结构里面放入\"弹出窗口\"这样的VI保证该循环畅通无阻。"
        n98 = event-data() -> ()  [unwired: 1 in, 1 out]
      }
      event Panel Close? {
        w255 = u16 1 items=["HPRI"=1, "LPRI"=0] ("priority")
        n99 = event-data() -> ()  [unwired: 1 in, 4 out]
        n100 = call "Enqueue Element Array.vi"("priority"=w255, "queue index"=0, "error in"=w259, "master data"="*Exit application", "queue in"=w260) -> ("error out"=w258:errorcluster, "queue out"=w257:T13)  [unwired: 5 in]
        n101 = event-data("Discard?"=TRUE) -> ()  [unwired: 1 in, 1 out]
      }
      event Value Change {
        w268 = u16 1 items=["HPRI"=1, "LPRI"=0] ("priority")
        n102 = event-data() -> ()  [unwired: 1 in, 6 out]
        n103 = call "Enqueue Element Array.vi"("priority"=w268, "queue index"=0, "error in"=w265, "master data"="Vision Paramter Save", "queue in"=w266) -> ("error out"=w263:errorcluster, "queue out"=w264:T13)  [unwired: 5 in]
      }
      event "取消按钮": Value Change {
        w275 = u16 1 items=["HPRI"=1, "LPRI"=0] ("priority")
        n104 = event-data() -> ()  [unwired: 1 in, 6 out]
        n105 = call "Enqueue Element Array.vi"("priority"=w275, "queue index"=0, "error in"=w272, "master data"="确认按钮", "queue in"=w273) -> ("error out"=w270:errorcluster, "queue out"=w271:T13)  [unwired: 5 in]
      }
      event "保存按钮": Value Change {
        w282 = u16 1 items=["HPRI"=1, "LPRI"=0] ("priority")
        n106 = event-data() -> ()  [unwired: 1 in, 6 out]
        n107 = call "Enqueue Element Array.vi"("priority"=w282, "queue index"=0, "error in"=w279, "master data"="程序参数保存", "queue in"=w280) -> ("error out"=w277:errorcluster, "queue out"=w278:T13)  [unwired: 5 in]
      }
      event "获取图像": Value Change {
        w290 = u16 1 items=["HPRI"=1, "LPRI"=0] ("priority")
        # "导丝上料位置范围设定参数"
        n108 = event-data() -> ()  [unwired: 1 in, 6 out]
        n109 = property on="Main" class="TabCtl (严格)"("Value"=enum32{"主参数", "模板匹配参数 ", "位置范围设定", "测试效果"}."测试效果" ("Main")) -> ()  [unwired: 2 in, 2 out]
        n110 = call "Enqueue Element Array.vi"("priority"=w290, "queue index"=0, "error in"=w287, "master data"="获取图像", "queue in"=w288) -> ("error out"=w285:errorcluster, "queue out"=w286:T13)  [unwired: 5 in]
      }
      event "保存图像": Value Change {
        w297 = u16 1 items=["HPRI"=1, "LPRI"=0] ("priority")
        n111 = event-data() -> ()  [unwired: 1 in, 6 out]
        n112 = call "Enqueue Element Array.vi"("priority"=w297, "queue index"=0, "error in"=w294, "master data"="保存图像", "queue in"=w295) -> ("error out"=w292:errorcluster, "queue out"=w293:T13)  [unwired: 5 in]
      }
      event "创建模板": Value Change {
        w304 = u16 1 items=["HPRI"=1, "LPRI"=0] ("priority")
        n113 = event-data() -> ()  [unwired: 1 in, 6 out]
        n114 = call "Enqueue Element Array.vi"("priority"=w304, "queue index"=0, "error in"=w301, "master data"="创建模板", "queue in"=w302) -> ("error out"=w299:errorcluster, "queue out"=w300:T13)  [unwired: 5 in]
      }
      event "ROI获取": Value Change {
        w312 = u16 1 items=["HPRI"=1, "LPRI"=0] ("priority")
        n115 = event-data() -> ()  [unwired: 1 in, 6 out]
        n116 = property on="Main" class="TabCtl (严格)"("Value"=enum32{"主参数", "模板匹配参数 ", "位置范围设定", "测试效果"}."模板匹配参数 " ("Main")) -> ()  [unwired: 2 in, 2 out]
        n117 = call "Enqueue Element Array.vi"("priority"=w312, "queue index"=0, "error in"=w309, "master data"="ROI获取", "queue in"=w310) -> ("error out"=w307:errorcluster, "queue out"=w308:T13)  [unwired: 5 in]
      }
      event "测试按钮": Value Change {
        w320 = u16 1 items=["HPRI"=1, "LPRI"=0] ("priority")
        n118 = event-data() -> ()  [unwired: 1 in, 6 out]
        n119 = call "Enqueue Element Array.vi"("priority"=w320, "queue index"=0, "error in"=w317, "master data"="测试按钮", "queue in"=w318) -> ("error out"=w315:errorcluster, "queue out"=w316:T13)  [unwired: 5 in]
        n120 = property on="Main" class="TabCtl (严格)"("Value"=enum32{"主参数", "模板匹配参数 ", "位置范围设定", "测试效果"}."测试效果" ("Main")) -> ()  [unwired: 2 in, 2 out]
      }
      event "刷新": Value Change {
        n121 = event-data() -> ()  [unwired: 1 in, 6 out]
        n122 = disable-structure shown="禁用" {
          disable-tunnel: w326 -> [w330 _]
          disable-tunnel: w325 -> [w329 _]
          disable-tunnel: [w328 _] -> w324
          disable-tunnel: [w327 _] -> w323
          frame Disabled {
            w332 = u16 1 items=["HPRI"=1, "LPRI"=0] ("priority")
            # "刷新"
            n123 = call "Enqueue Element Array.vi"("priority"=w332, "queue index"=0, "error in"=w329, "master data"="刷新", "queue in"=w330) -> ("error out"=w327:errorcluster, "queue out"=w328:T13)  [unwired: 5 in]
          }
          frame Enabled {
          }
        }
        n124 = property on="Main" class="TabCtl (严格)"("Value"=enum32{"主参数", "模板匹配参数 ", "位置范围设定", "测试效果"}."模板匹配参数 " ("Main")) -> ()  [unwired: 2 in, 2 out]
      }
    }
    n125 = call "GetSystemTime.vi"() -> ("date/time string"=→"system time":string)  [unwired: 7 in]
  }
  n126 = call "Release Queue Array.vi"("error in"=w3, "queue in"=w1) -> ("error out"=w2:errorcluster)  [unwired: 2 in, 3 out]
  n127 = call "Release Queue Array.vi"("error in"=w6, "queue in"=w1) -> ("error out"=w9:errorcluster)  [unwired: 2 in, 3 out]
  n128 = call "MergeErrors.vi"("error in 3 (no error)"=w2, "error in 4 (no error)"=w9) -> ("error out"=w8:errorcluster)  [unwired: 6 in]
  n129 = call "ExitAppMode.vi"("error in (no error)"=w8) -> ("error out"=w7:errorcluster)  [unwired: 10 in]
  n130 = call <vilib>:"Clear Errors.vi"("error in (no error)"=w7) -> ()  [unwired: 5 in, 2 out]
